vi "Joystick Controls.vi"() -> (3 "Input Cluster":T1)   [LabVIEW 2015]
uses:
  Joytsick/Joytstick Controls Type.ctl
  Global Vars.vi
  <vilib>/Rock Robotics/WPI/Utilities/WPI_GetSetVariantRefNum.vi
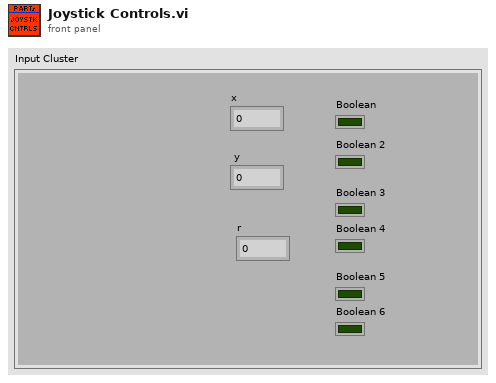
[diagram p1: front panel]
types:
  T1 = typedef "Joytstick Controls Type.ctl" = cluster{"x":dbl, " y":dbl, "r":dbl, "Boolean":bool, "Boolean 2":bool, "Boolean 3":bool, "Boolean 4":bool, "Boolean 5":bool, "Boolean 6":bool}
  T2 = typedef "WPI_JoystickDevRef.ctl" = cluster{"Device":T3}
  T3 = typedef "WPI_JoystickDeviceEnum.ctl" = enum16{"USB 0", "USB 1", "USB 2", "USB 3", "USB 4", "USB 5"}
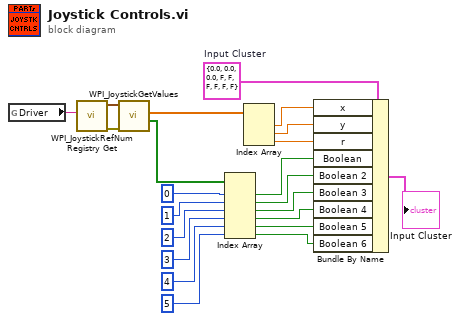
[diagram p0: block diagram]
diagram:
  w10 = T1 {"x"=0.0, " y"=0.0, "r"=0.0, "Boolean"=FALSE, "Boolean 2"=FALSE, "Boolean 3"=FALSE, "Boolean 4"=FALSE, "Boolean 5"=FALSE, "Boolean 6"=FALSE}  # Input Cluster
  n1 = global read "Global Vars.vi" "Driver"() -> (w21:string)
  n2 = call <vilib>:"WPI_JoystickRefNum Registry Get.vi"("refnum name"=w21) -> ("error out"=w19:errorcluster, "JoystickDevRef"=w20:T2)  [unwired: 9 in]
  n3 = call <vilib>:"WPI_JoystickGetValues.vi"("error in (no error)"=w19, "JoystickDevRef"=w20) -> ("Buttons"=w18:bool[], "Axes"=w22:dbl[])  [unwired: 5 in, 3 out]
  n4 = Index Array(array=w18, index #1=0 ("index"), index #2=1 ("index"), index #3=2 ("index"), index #4=3 ("index"), index #5=4 ("index"), index #6=5 ("index")) -> (element #1=w9:bool, element #2=w8:bool, element #3=w7:bool, element #4=w6:bool, element #5=w5:bool, element #6=w1:bool)
  n5 = Index Array(array=w22) -> (element #1=w17:dbl, element #2=w16:dbl, element #3=w15:dbl)  [unwired: 3 in]
  n6 = Bundle By Name(cluster=w10, "x"=w17, "y"=w16, "r"=w15, "Boolean"=w9, "Boolean 2"=w8, "Boolean 3"=w7, "Boolean 4"=w6, "Boolean 5"=w5, "Boolean 6"=w1) -> (→"Input Cluster":T1)
